vi "4.vi"() -> ()   [LabVIEW 2019]
panel:
  out "Iteration Count":dbl
  in  "Stop":bool
  out "Output":dbl
  in  "Operation":enum16{"Add", "Subtract", "Multiply", "Divide"}(ring)
  in  "B":dbl
  in  "A":dbl
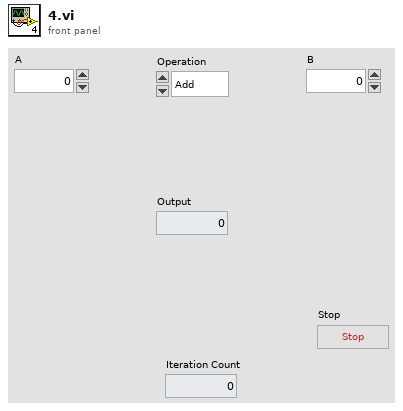
[diagram p1: front panel]
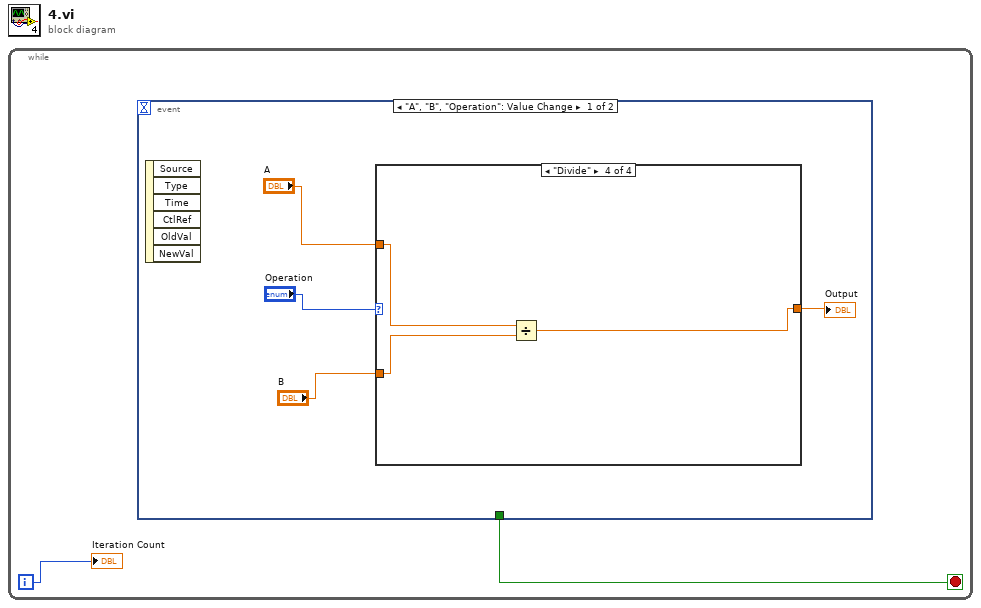
[diagram p0: block diagram]
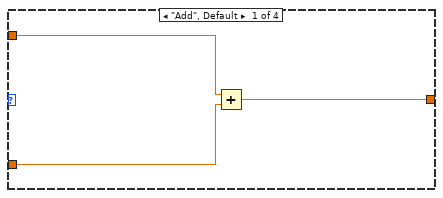
[diagram p2: hidden frame]
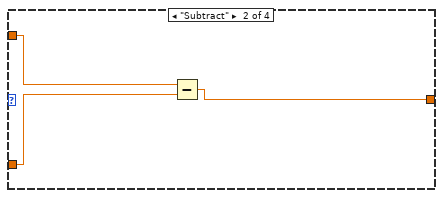
[diagram p3: hidden frame]
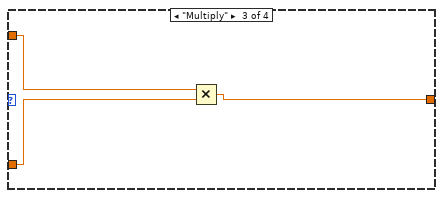
[diagram p4: hidden frame]
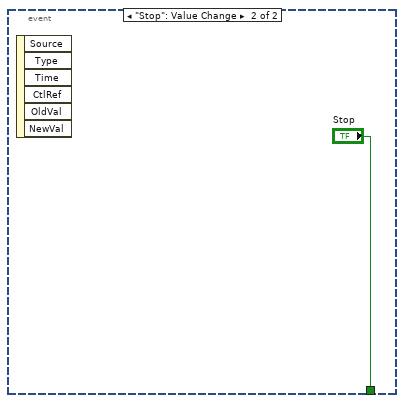
[diagram p5: hidden frame]
diagram:
  n1 = while {
    i -> [w1]
    stop <- w2 stop-if-true
    n2 = event shown="[0] \"A\", \"B\", \"Operation\": Value Change" {
      selector: _ -> [_ _]
      dyn-events: _ -> [_ _]
      timeout: _ -> [_ _]
      tunnel: [_ "Stop"] -> w2
      event "A", "B", "Operation": Value Change {
        n3 = event-data() -> ()  [unwired: 1 in, 6 out]
        n4 = case shown="\"Divide\"" "Operation" {
          tunnel: "A" -> [w9 w12 w15 w18]
          tunnel: "B" -> [w8 w11 w14 w17]
          tunnel: [w7 w10 w13 w16] -> w4
          frame "Add", Default {
            n5 = Add(x=w9, y=w8) -> (x+y=w7:dbl)
          }
          frame "Subtract" {
            n6 = Subtract(x=w12, y=w11) -> (x-y=w10:dbl)
          }
          frame "Multiply" {
            n7 = Multiply(x=w15, y=w14) -> (x*y=w13:dbl)
          }
          frame "Divide" {
            n8 = Divide(x=w18, y=w17) -> (x/y=w16:dbl)
          }
        }
        "Output" <- w4
      }
      event "Stop": Value Change {
        n9 = event-data() -> ()  [unwired: 1 in, 6 out]
      }
    }
    "Iteration Count" <- w1
  }
